vi "createMissionWaypoints.vi"(8 "error in (no error)":errorcluster, 11 "RoundBuoy in":refnum<class "RoundBuoy.lvclass">) -> (0 "error out":errorcluster, 3 "RoundBuoy out":refnum<class "RoundBuoy.lvclass">)   [LabVIEW 2011, in "RoundBuoy.lvclass"]
uses:
  RoundBuoy.lvclass
  Waypoint/Waypoint.lvclass
  2 Globals/2 Global.vi
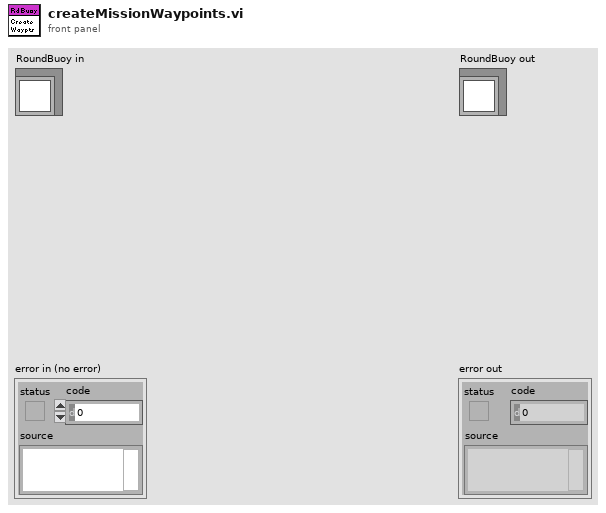
[diagram p1: front panel]
types:
  T1 = typedef "UTM Location.ctl" = cluster{"UTM Zone":dbl, "Hemisphere":enum16{"North", "South"}, "East":dbl, "North":dbl}
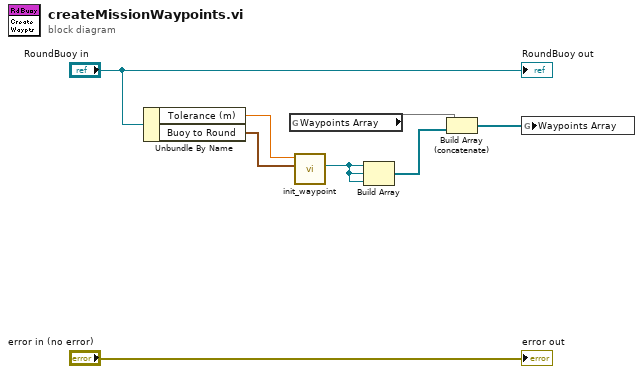
[diagram p0: block diagram]
diagram:
  n1 = Unbundle By Name("RoundBuoy in") -> ("Tolerance (m)"=w8:dbl, "Buoy to Round"=w1:T1)
  n2 = global read "2 Global.vi" "Waypoints Array"() -> (w6)
  n3 = call "init_waypoint.vi"("Coords"=w1, "Tolerance (m)"=w8) -> ("Waypoint Out"=w7:refnum<class "Waypoint.lvclass">)  [unwired: 9 in]
  n4 = Build Array(w7, w7, w7) -> (w5:refnum<class "Waypoint.lvclass">[])
  n5 = Build Array (concatenate)(w6, w5) -> (w4:refnum<class "Waypoint.lvclass">[])
  n6 = global write "2 Global.vi" "Waypoints Array"(w4) -> ()
  "error out" <- "error in (no error)"
  "RoundBuoy out" <- "RoundBuoy in"
